vi "Read TestResultInformation.vi"(8 "error in (no error)":errorcluster, 11 "TestResultInformation in":refnum<class "TestResultInformation.lvclass">) -> (0 "error out":errorcluster, 2 "TestResultInformation":T1, 3 "TestResultInformation out":refnum<class "TestResultInformation.lvclass">)   [LabVIEW 2019, in "TestEngine.lvlib" / "TestResultInformation.lvclass"]
uses:
  TestResultInformation.lvclass
  TestResultInformation.lvclass/TestResultInformation.ctl
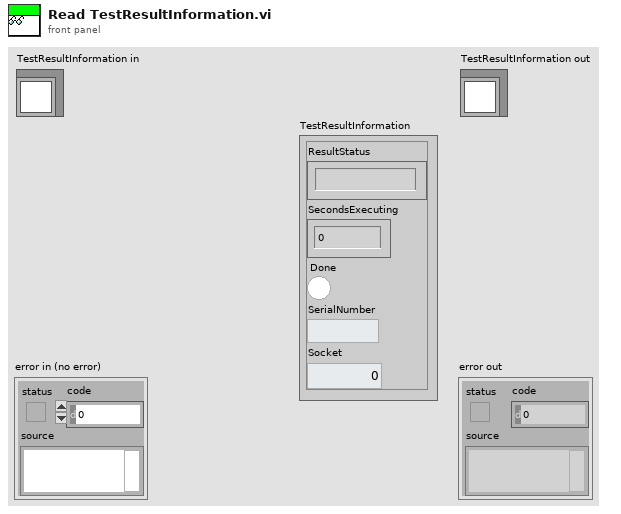
[diagram p1: front panel]
types:
  T1 = cluster{"ResultStatus":string, "SecondsExecuting":dbl, "Done":bool, "SerialNumber":string, "Socket":i32}
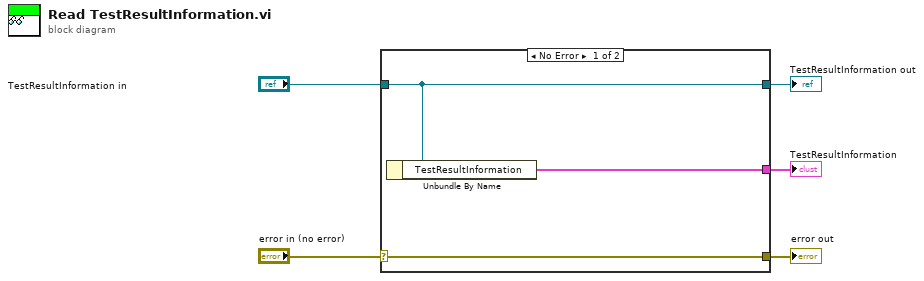
[diagram p0: block diagram]
diagram:
  n1 = case shown="No Error" "error in (no error)" {
    selector: "error in (no error)" -> [w8 w9]
    tunnel: [w8 w9] -> w4
    tunnel: [w7 w10] -> w2
    tunnel: "TestResultInformation in" -> [w7 w10]
    tunnel: [w6 _] -> w1
    frame No Error {
      n2 = Unbundle By Name(w7) -> ("TestResultInformation"=w6:T1)
    }
    frame Error {
    }
  }
  "error out" <- w4
  "TestResultInformation out" <- w2
  "TestResultInformation" <- w1
